vi "CRYData View Legend Item Insert.vi"(8 "Item Symbols":i32[](array[numeric]), 9 "Color Array":u32[](array[colorbox]), 10 "ItemName Array":string[](array[string]), 11 "Legend MultiListbox":refnum<vi>) -> ()   [LabVIEW 2013]
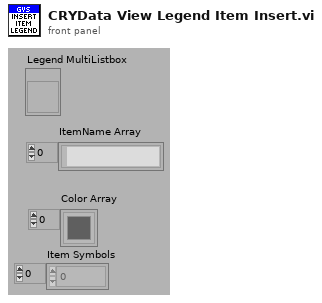
[diagram p1: front panel]
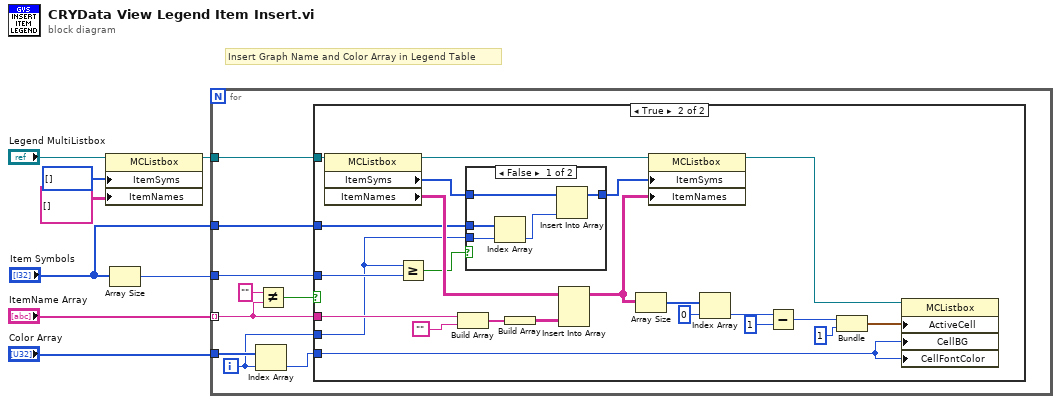
[diagram p0: block diagram]
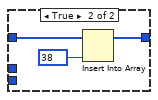
[diagram p3: hidden frame]
diagram:
  # "Insert Graph Name and Color Array in Legend Table"
  n1 = property on="Property Node" class="MCListbox"(reference="Legend MultiListbox", "ItemSyms"=i32[] [] ("Item Symbols"), "ItemNames"=string[][] [] ("Item Names")) -> (reference out=w5:refnum<vi>)  [unwired: 1 in, 1 out]
  n2 = Array Size(array="Item Symbols") -> (size(s)=w3:i32)
  n3 = for {
    tunnel: w5 -> [w17]
    tunnel: "Color Array" -> [w11]
    tunnel: "ItemName Array" -> [w15] mode=indexing
    tunnel: w3 -> [w13]
    tunnel: "Item Symbols" -> [w12]
    i -> [w10]
    n4 = Index Array(array=w11, index=w10) -> (element=w9:u32)
    n5 = Not Equal?(x="", y=w15) -> (x != y?=w16:bool)
    n6 = case shown="True" w16 {
      tunnel: w17 -> [_ w40]
      tunnel: w9 -> [_ w22]
      tunnel: w15 -> [_ w25]
      tunnel: w13 -> [_ w21]
      tunnel: w10 -> [_ w18]
      tunnel: w12 -> [_ w19]
      frame False {
      }
      frame True {
        n7 = property on="Property Node" class="MCListbox"(reference=w40) -> (reference out=w39:refnum<vi>, "ItemSyms"=w38:i32[], "ItemNames"=w36:string[][])  [unwired: 1 in, 1 out]
        n8 = Greater Or Equal?(x=w18, y=w21) -> (x >= y?=w20:bool)
        n9 = Build Array(w25, "") -> (w24:string[])
        n10 = case shown="False" w20 {
          tunnel: w38 -> [w45 w48]
          tunnel: [w44 w47] -> w37
          tunnel: w19 -> [w43 _]
          tunnel: w18 -> [w42 _]
          frame False {
            n11 = Index Array(array=w43, index=w42) -> (element=w41:i32)
            n12 = Insert Into Array(array=w45, new element=w41) -> (w44:i32[])  [unwired: 1 in]
          }
          frame True {
            n13 = Insert Into Array(array=w48, new element=38) -> (w47:i32[])  [unwired: 1 in]
          }
        }
        n14 = Build Array(w24) -> (w23:string[][])
        n15 = Insert Into Array(array=w36, new element=w23) -> (w35:string[][])  [unwired: 2 in]
        n16 = Array Size(array=w35) -> (size(s)=w34:i32[])
        n17 = property on="Property Node" class="MCListbox"(reference=w39, "ItemSyms"=w37, "ItemNames"=w35) -> (reference out=w27:refnum<vi>)  [unwired: 1 in, 1 out]
        n18 = Index Array(array=w34, index=0) -> (element=w32:i32)
        n19 = Subtract(x=w32, y=1) -> (x-y=w30:i32)
        n20 = Bundle(w30, "y"=1) -> (w28:cluster{i32, "y":i32})  [unwired: 1 out]
        n21 = property class="MCListbox"(reference=w27, "ActiveCell"=w28, "CellBG"=w22, "CellFontColor"=w22) -> ()  [unwired: 1 in, 2 out]
      }
    }
  }
